vi "progra 8.vi"() -> ()   [LabVIEW 2011]
panel:
  out "Contador":dbl
  out "Temp 36-60":dbl
  out "Temp 21-35":dbl
  out "Temp 1-20":dbl
  out "Temperatura":i32(slide) scale=0.0..60.0
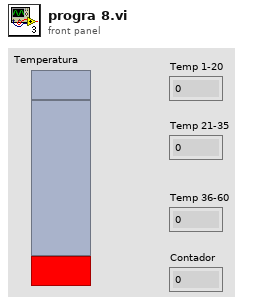
[diagram p1: front panel]
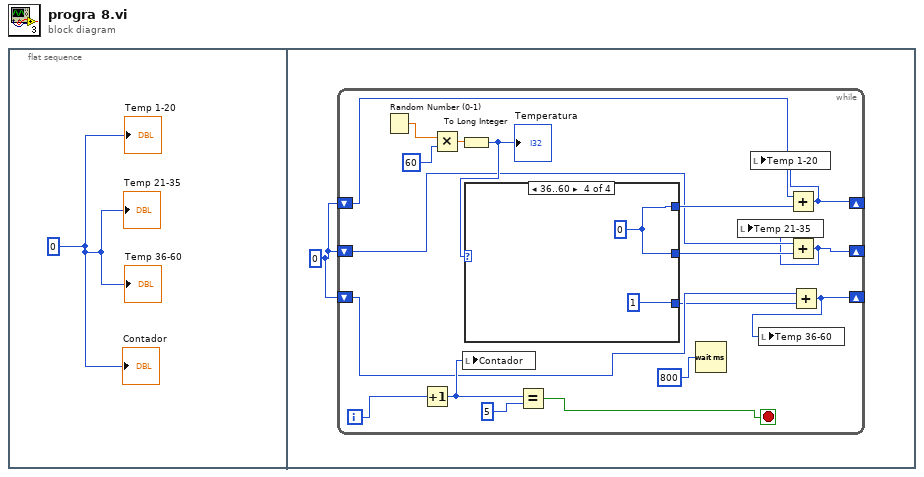
[diagram p0: block diagram]
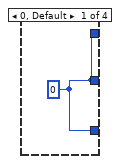
[diagram p2: hidden frame]
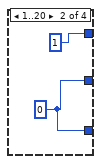
[diagram p3: hidden frame]
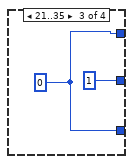
[diagram p4: hidden frame]
diagram:
  n1 = flat-sequence {
    frame #0 {
      w1 = 0
      "Temp 1-20" <- w1
      "Temp 21-35" <- w1
      "Temp 36-60" <- w1
      "Contador" <- w1
    }
    frame #1 {
      w2 = 0
      n2 = while {
        shift-right: [w5] -> _
        shift-left: w2 -> [w11]
        shift-right: [w4] -> _
        shift-left: w2 -> [w9]
        shift-right: [w3] -> _
        shift-left: w2 -> [w7]
        i -> [w18]
        stop <- w15 stop-if-true
        n3 = Random Number (0-1)() -> (number: 0 to 1=w19:dbl)
        n4 = Increment(x=w18) -> (x+1=w16:i32)
        n5 = Multiply(x=w19, y=60) -> (x*y=w13:dbl)
        n6 = To Long Integer(number=w13) -> (32bit integer=w12:i32)
        "Temperatura" <- w12
        n7 = local write "Contador"(w16) -> ()
        n8 = case shown="36..60" w12 {
          tunnel: [w21 1 w25 w27] -> w10
          tunnel: [w21 w23 1 w27] -> w8
          tunnel: [w21 w23 w25 1] -> w6
          frame 0, Default {
            w21 = 0
          }
          frame 1..20 {
            w23 = 0
          }
          frame 21..35 {
            w25 = 0
          }
          frame 36..60 {
            w27 = 0
          }
        }
        n9 = Equal?(x=w16, y=5) -> (x = y?=w15:bool)
        n10 = Wait (ms)(milliseconds to wait=800) -> ()  [unwired: 1 out]
        n11 = Add(x=w11, y=w10) -> (x+y=w5:i32)
        n12 = local write "Temp 1-20"(w5) -> ()
        n13 = Add(x=w9, y=w8) -> (x+y=w4:i32)
        n14 = local write "Temp 21-35"(w4) -> ()
        n15 = Add(x=w7, y=w6) -> (x+y=w3:i32)
        n16 = local write "Temp 36-60"(w3) -> ()
      }
    }
  }
